vi "ABR-Restore Defaults.vi"() -> (4 "Params":T1={"CAP or ABR"=enum."ABR", "Stimulus"={"Destination"="", "Waveform"=enum."TONE PIP", "Frequency (kHz)"=16.0, "Rep rate (/sec)"=30.0, "Alternate Polarity"=FALSE, "Sampling rate (Hz)"=0.0, "Duration (ms)"=30.0, "Ramp (ms)"=5.0, "Click width (us)"=0.0, "ITI"=enum."Rate", "Save raw"=FALSE}, "Sequence"={"Start (dB)"=25000, "Stop (dB)"=100000, "Step (dB)"=5}, "Response"={"Gain"=10000, "Averages"=512, "Window (ms)"=8.5, "Thr Fast Steps"=8.5, "Sampling rate (Hz)"=25000.0}} {"Sequence"."Start (dB)" step=5; "Response"."Thr Fast Steps" format="%.2f"; "Response"."Window (ms)" format="%.2f"; "Stimulus"."Frequency (kHz)" format="%.2f"}, 8 "Threshold Estimation":T5={"Tmin (ms)"=0.0, "Tmax (ms)"=8.5, "CC criterion"=0.35, "adjR2 criterion"=0.7}, 15 "error out":errorcluster)   [LabVIEW 2020]
uses:
  Typedefs/ABR-Parameters.ctl
  Typedefs/ABR-Stimulus.ctl
  Typedefs/ABR-Sequence.ctl
  Typedefs/ABR-Response.ctl
  Threshold Estimation VIs/ABR3-Threshold Estimation Parameters.ctl
  Typedefs/ABR-Legacy Parameters.ctl
  2fda9144-15ab-4c0b-9eae-791234703d3e.vi
panel:
  in  "Defaults":T1={"CAP or ABR"=enum."ABR", "Stimulus"={"Destination"="Right", "Waveform"=enum."TONE PIP", "Frequency (kHz)"=16.0, "Rep rate (/sec)"=30.0, "Alternate Polarity"=TRUE, "Sampling rate (Hz)"=100000.0, "Duration (ms)"=5.0, "Ramp (ms)"=5.0, "Click width (us)"=0.0, "ITI"=enum."Rate", "Save raw"=FALSE}, "Sequence"={"Start (dB)"=20, "Stop (dB)"=80, "Step (dB)"=5}, "Response"={"Gain"=10000, "Averages"=512, "Window (ms)"=8.5, "Thr Fast Steps"=1.5, "Sampling rate (Hz)"=25000.0}} {"Sequence"."Start (dB)" step=5; "Response"."Thr Fast Steps" format="%.2f"; "Response"."Window (ms)" format="%.2f"; "Stimulus"."Frequency (kHz)" format="%.2f"}
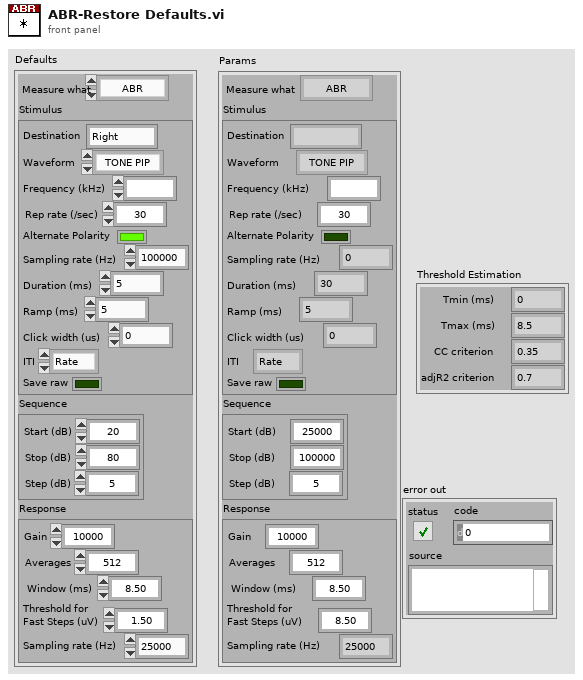
[diagram p1: front panel]
types:
  T1 = typedef "ABR-Parameters.ctl" = cluster{"CAP or ABR":enum16{"CAP", "ABR"}, "Stimulus":T2, "Sequence":T3, "Response":T4}
  T2 = typedef "ABR-Stimulus.ctl" = cluster{"Destination":string, "Waveform":enum16{"TONE PIP", "CLICK"}, "Frequency (kHz)":ext, "Rep rate (/sec)":dbl, "Alternate Polarity":bool, "Sampling rate (Hz)":dbl, "Duration (ms)":dbl, "Ramp (ms)":dbl, "Click width (us)":dbl, "ITI":enum16{"Rate", "Interval"}, "Save raw":bool}
  T3 = typedef "ABR-Sequence.ctl" = cluster{"Start (dB)":i32, "Stop (dB)":i32, "Step (dB)":i32}
  T4 = typedef "ABR-Response.ctl" = cluster{"Gain":i32, "Averages":i32, "Window (ms)":sgl, "Thr Fast Steps":sgl, "Sampling rate (Hz)":dbl}
  T5 = typedef "ABR3-Threshold Estimation Parameters.ctl" = cluster{"Tmin (ms)":dbl, "Tmax (ms)":dbl, "CC criterion":dbl, "adjR2 criterion":dbl}
  T6 = typedef "ABR-Legacy Parameters.ctl" = cluster{"CAP or ABR":enum16{"CAP", "ABR"}, "Stimulus":cluster{"Ear":enum16{"Right", "Left", "Bone"}, "Start (dB)":i32, "Waveform":enum16{"TONE PIP", "CLICK"}, "Stop (dB)":i32, "Frequency (kHz)":ext, "Step (dB)":i32, "Rep rate (/sec)":dbl, "Alternate Polarity":bool}, "Response":cluster{"Gain":i32, "Averages":i32, "Window (ms)":sgl, "Thr Fast Steps":sgl}, "Hidden":cluster{"AI Samp Rate Hz":dbl, "AO Samp Rate Hz":dbl, "Duration (ms)":dbl, "Ramp (ms)":dbl, "Click width (us)":dbl, "ITI":enum16{"Rate", "Interval"}, "Save raw":bool}, "Version":i32}
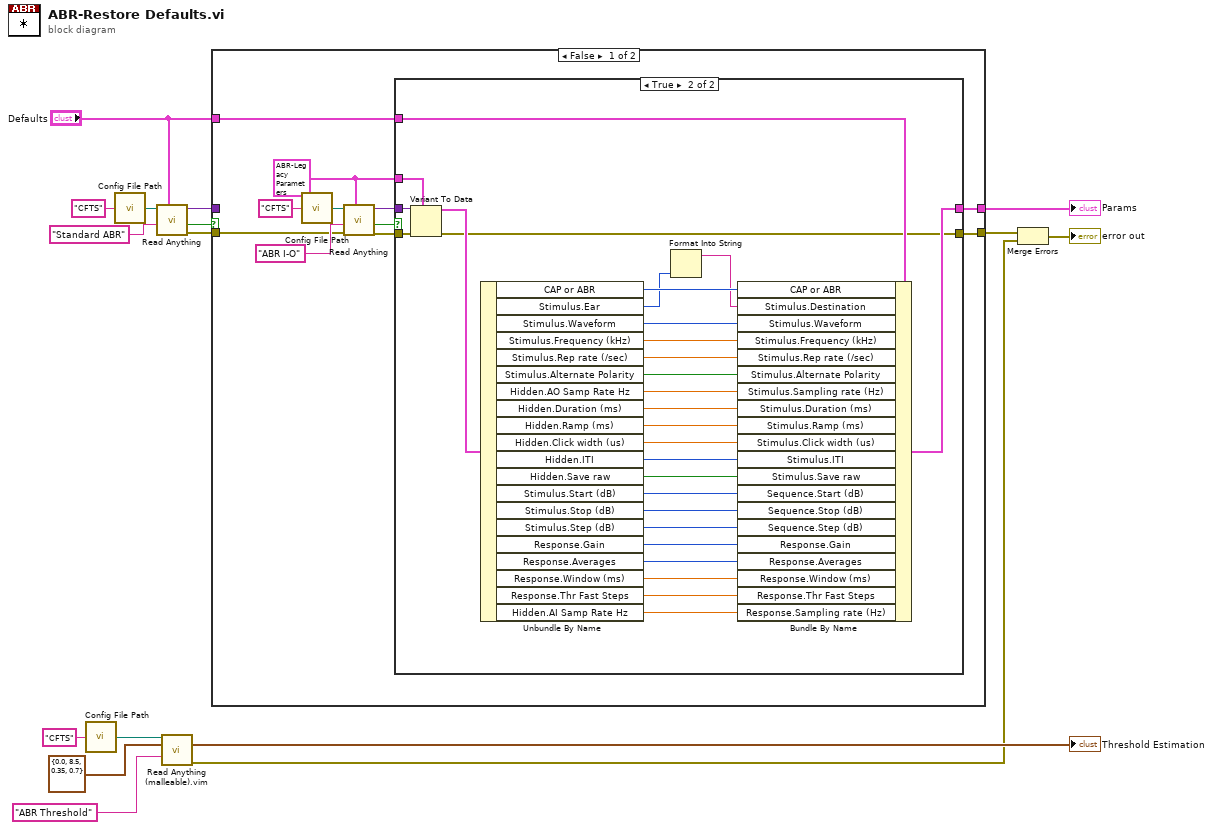
[diagram p0: block diagram]
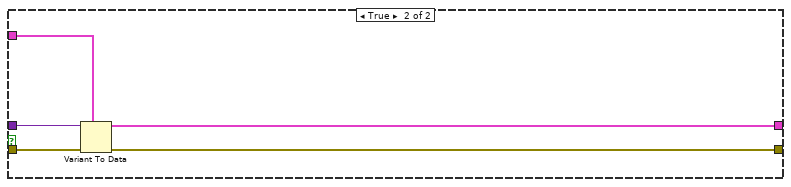
[diagram p3: hidden frame]
diagram:
  n1 = call "Config File Path.vi"("AppName"="CFTS") -> ("Default config file name"=w8:path)
  n2 = call "Config File Path.vi"("AppName"="CFTS") -> ("Default config file name"=w6:path)
  n3 = call "Read Anything.vi"("Type of Anything"="Defaults", "Section Name (Name of \"Type of Anything\")"="Standard ABR" ("Section Name (Name of \"Type of Anything\")"), "Path (dialog)"=w6) -> ("Error Out"=w14:errorcluster, "Found?"=w13:bool, "Anything"=w16:variant)  [unwired: 6 in]
  n4 = call "Read Anything (malleable).vim"("Config file path"=w8, "Options in"=T5 {"Tmin (ms)"=0.0, "Tmax (ms)"=8.5, "CC criterion"=0.35, "adjR2 criterion"=0.7} ("Threshold Estimation"), "Section"="ABR Threshold" ("Section Name (Name of \"Type of Anything\")")) -> ("Options out"=→"Threshold Estimation":T5, "error out"=w2:errorcluster)  [unwired: 10 in, 1 out]
  n5 = case shown="False" w13 {
    tunnel: w16 -> [_ w62]
    tunnel: "Defaults" -> [w22 w61]
    tunnel: w14 -> [w23 w60]
    tunnel: [w27 w59] -> w4
    tunnel: [w17 w58] -> w3
    frame False {
      w19 = T6 {"CAP or ABR"=enum."ABR", "Stimulus"={"Ear"=enum."Left", "Start (dB)"=0, "Waveform"=enum."TONE PIP", "Stop (dB)"=30, "Frequency (kHz)"=16.0, "Step (dB)"=5, "Rep rate (/sec)"=30.0, "Alternate Polarity"=FALSE}, "Response"={"Gain"=10000, "Averages"=512, "Window (ms)"=8.5, "Thr Fast Steps"=8.5}, "Hidden"={"AI Samp Rate Hz"=25000.0, "AO Samp Rate Hz"=100000.0, "Duration (ms)"=5.0, "Ramp (ms)"=0.5, "Click width (us)"=0.0, "ITI"=enum."Rate", "Save raw"=FALSE}, "Version"=0} ("Params")
      n6 = call "Config File Path.vi"("AppName"="CFTS") -> ("Default config file name"=w24:path)
      n7 = call "Read Anything.vi"("Type of Anything"=w19, "Error In"=w23, "Section Name (Name of \"Type of Anything\")"="ABR I-O" ("Section Name (Name of \"Type of Anything\")"), "Path (dialog)"=w24) -> ("Error Out"=w20:errorcluster, "Found?"=w18:bool, "Anything"=w21:variant)  [unwired: 5 in]
      n8 = case shown="True" w18 {
        tunnel: [w29 w57] -> w27
        tunnel: w22 -> [w29 w56]
        tunnel: w21 -> [_ w55]
        tunnel: w20 -> [w28 w54]
        tunnel: w19 -> [_ w53]
        tunnel: [w28 w30] -> w17
        frame False {
        }
        frame True {
          n9 = Variant To Data(error in=w54, type=w53, Variant=w55) -> (data=w52:T6, error out=w30:errorcluster)
          n10 = Unbundle By Name(w52) -> ("CAP or ABR"=w51:enum16{"CAP", "ABR"}, "Stimulus.Ear"=w50:enum16{"Right", "Left", "Bone"}, "Stimulus.Waveform"=w48:enum16{"TONE PIP", "CLICK"}, "Stimulus.Frequency (kHz)"=w47:ext, "Stimulus.Rep rate (/sec)"=w46:dbl, "Stimulus.Alternate Polarity"=w45:bool, "Hidden.AO Samp Rate Hz"=w44:dbl, "Hidden.Duration (ms)"=w43:dbl, "Hidden.Ramp (ms)"=w42:dbl, "Hidden.Click width (us)"=w41:dbl, "Hidden.ITI"=w40:enum16{"Rate", "Interval"}, "Hidden.Save raw"=w39:bool, "Stimulus.Start (dB)"=w38:i32, "Stimulus.Stop (dB)"=w37:i32, "Stimulus.Step (dB)"=w36:i32, "Response.Gain"=w35:i32, "Response.Averages"=w34:i32, "Response.Window (ms)"=w33:sgl, "Response.Thr Fast Steps"=w32:sgl, "Hidden.AI Samp Rate Hz"=w31:dbl)
          n11 = Format Into String(w50) -> (resulting string=w49:string)  [unwired: 3 in, 1 out]
          n12 = Bundle By Name(cluster=w56, "CAP or ABR"=w51, "Stimulus.Destination"=w49, "Stimulus.Waveform"=w48, "Stimulus.Frequency (kHz)"=w47, "Stimulus.Rep rate (/sec)"=w46, "Stimulus.Alternate Polarity"=w45, "Stimulus.Sampling rate (Hz)"=w44, "Stimulus.Duration (ms)"=w43, "Stimulus.Ramp (ms)"=w42, "Stimulus.Click width (us)"=w41, "Stimulus.ITI"=w40, "Stimulus.Save raw"=w39, "Sequence.Start (dB)"=w38, "Sequence.Stop (dB)"=w37, "Sequence.Step (dB)"=w36, "Response.Gain"=w35, "Response.Averages"=w34, "Response.Window (ms)"=w33, "Response.Thr Fast Steps"=w32, "Response.Sampling rate (Hz)"=w31) -> (w57:T1)
        }
      }
    }
    frame True {
      n13 = Variant To Data(error in=w60, type=w61, Variant=w62) -> (data=w59:T1, error out=w58:errorcluster)
    }
  }
  "Params" <- w4
  n14 = Merge Errors(w3, w2) -> (→"error out":errorcluster)
